vi "Run Bitfile velocity.vi"() -> ()   [LabVIEW 2011]
uses:
  <vilib>/Platform/TimedLoop/XDataNode/timing_clust.ctl
  <vilib>/Platform/TimedLoop/XDataNode/nitl_modes.ctl
  <vilib>/Platform/TimedLoop/XDataNode/wakeup.ctl
  <vilib>/FPGAPlugInAG/sbRIO-9606/niLvFpga_Open_sbRIO-9606.vi
  <vilib>/rvi/interface/common/dynamic/niFpgaDynamicAddResources.vi
  <vilib>/Utility/error.llb/Error Cluster From Error Code.vi
  <vilib>/rvi/errors/niLvFpgaAdjustHostInterfaceError.vi
  <vilib>/FPGAPlugInAG/Dynamic/niLvFpga_Close_Dynamic.vi
  <vilib>/Platform/TimedLoop/XDataNode/XDataNode.xnode
  <vilib>/rvi/interface/nirviOpenFPGA/nirviOpenFPGA.xnode
  labview/FPGA Bitfiles/natcar_FPGATarget_Top-Level_610FB000.lvbitx
  <vilib>/rvi/interface/nirviReadWriteControl/nirviReadWriteControl.xnode
  <vilib>/rvi/interface/nirviCloseFPGA/nirviCloseFPGA.xnode
  <vilib>/Platform/TimedLoop/XDataNode/XDNodeRunTimeDep.lvlib
  NiFpgaLv.dll
  <vilib>/rvi/interface/Simulation/niFpgaSimulationCallBeginRW.vi
panel:
  out "Speed Error":dbl(graph)
  in  "Offset":dbl=22.0 min=0.0 max=30.0 step=0.1
  out "Velocity counts":u32
  out "V [m/s]":dbl
  in  "RUN!":bool
  in  "Stop":bool
  in  "Kff":dbl=6.0 min=0.0 max=10.0 step=0.1
  in  "uBlaze Reset":bool
  in  "Steering ON 1e-7s":u32=15000 min=10240 max=19650 step=100
  in  "Steering":bool
  in  "Throttle":bool
  in  "GO frequency (Hz)":u16=1000 min=10 max=10000 step=10
  in  "GO duty (100*%)":u16 max=100 step=1
  in  "V desired [m/s]":dbl min=0.0 max=5.0 step=0.1
  in  "Speed Ki":dbl=0.1 min=0.0 max=2.0 step=0.01
  in  "Throttle ON":bool
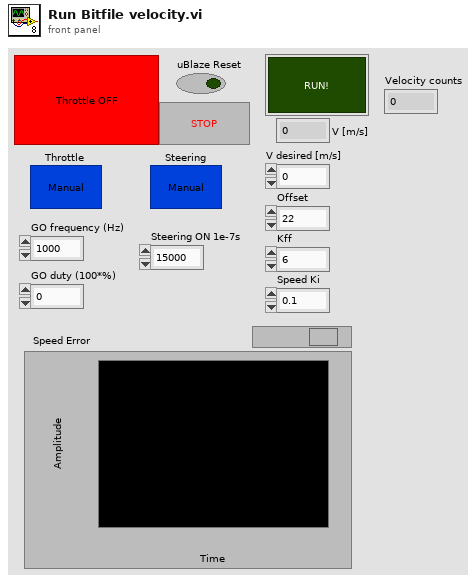
[diagram p1: front panel]
types:
  T1 = typedef "XDNodeRunTimeDep.lvlib/timing_clust.ctl" = cluster{"Expected End [f-1]":u64, "Actual End [f-1]":u64, "Finished Late? [f-1]":bool, "Expected End [i-1]":u64, "Actual End [i-1]":u64, "Finished Late? [i-1]":bool, "Expected Start [i]":u64, "Actual Start [i]":u64, "Expected Start [f]":u64, "Actual Start [f]":u64, "Source Name":string, "Structure Name":string, "Period":i64, "Deadline":i64, "Offset":i64, "Start":i64, "Priority":i32, "Timeout":i32, "Mode":T2, "Wakeup Reason":T3, "Error":errorcluster, "Source Type":string, "Secondary Source Type":string, "Global End Time":u64, "Global Start Time":u64, "Frame Duration":u64, "Iteration Duration":u64, "Assigned CPU":i32, "I/O Scan Engine Mode":u32}
  T2 = typedef "XDNodeRunTimeDep.lvlib/nitl_modes.ctl" = enum32{"No Change", "Process missed periods, maintain original phase", "Discard missed periods, maintain original phase", "Process missed periods, ignore original phase", "Discard missed periods, ignore original phase"}
  T3 = typedef "XDNodeRunTimeDep.lvlib/wakeup.ctl" = enum32{"Normal", "Aborted", "Asynchronous wakeup", "Timing source error", "Timed loop error", "Timeout"}
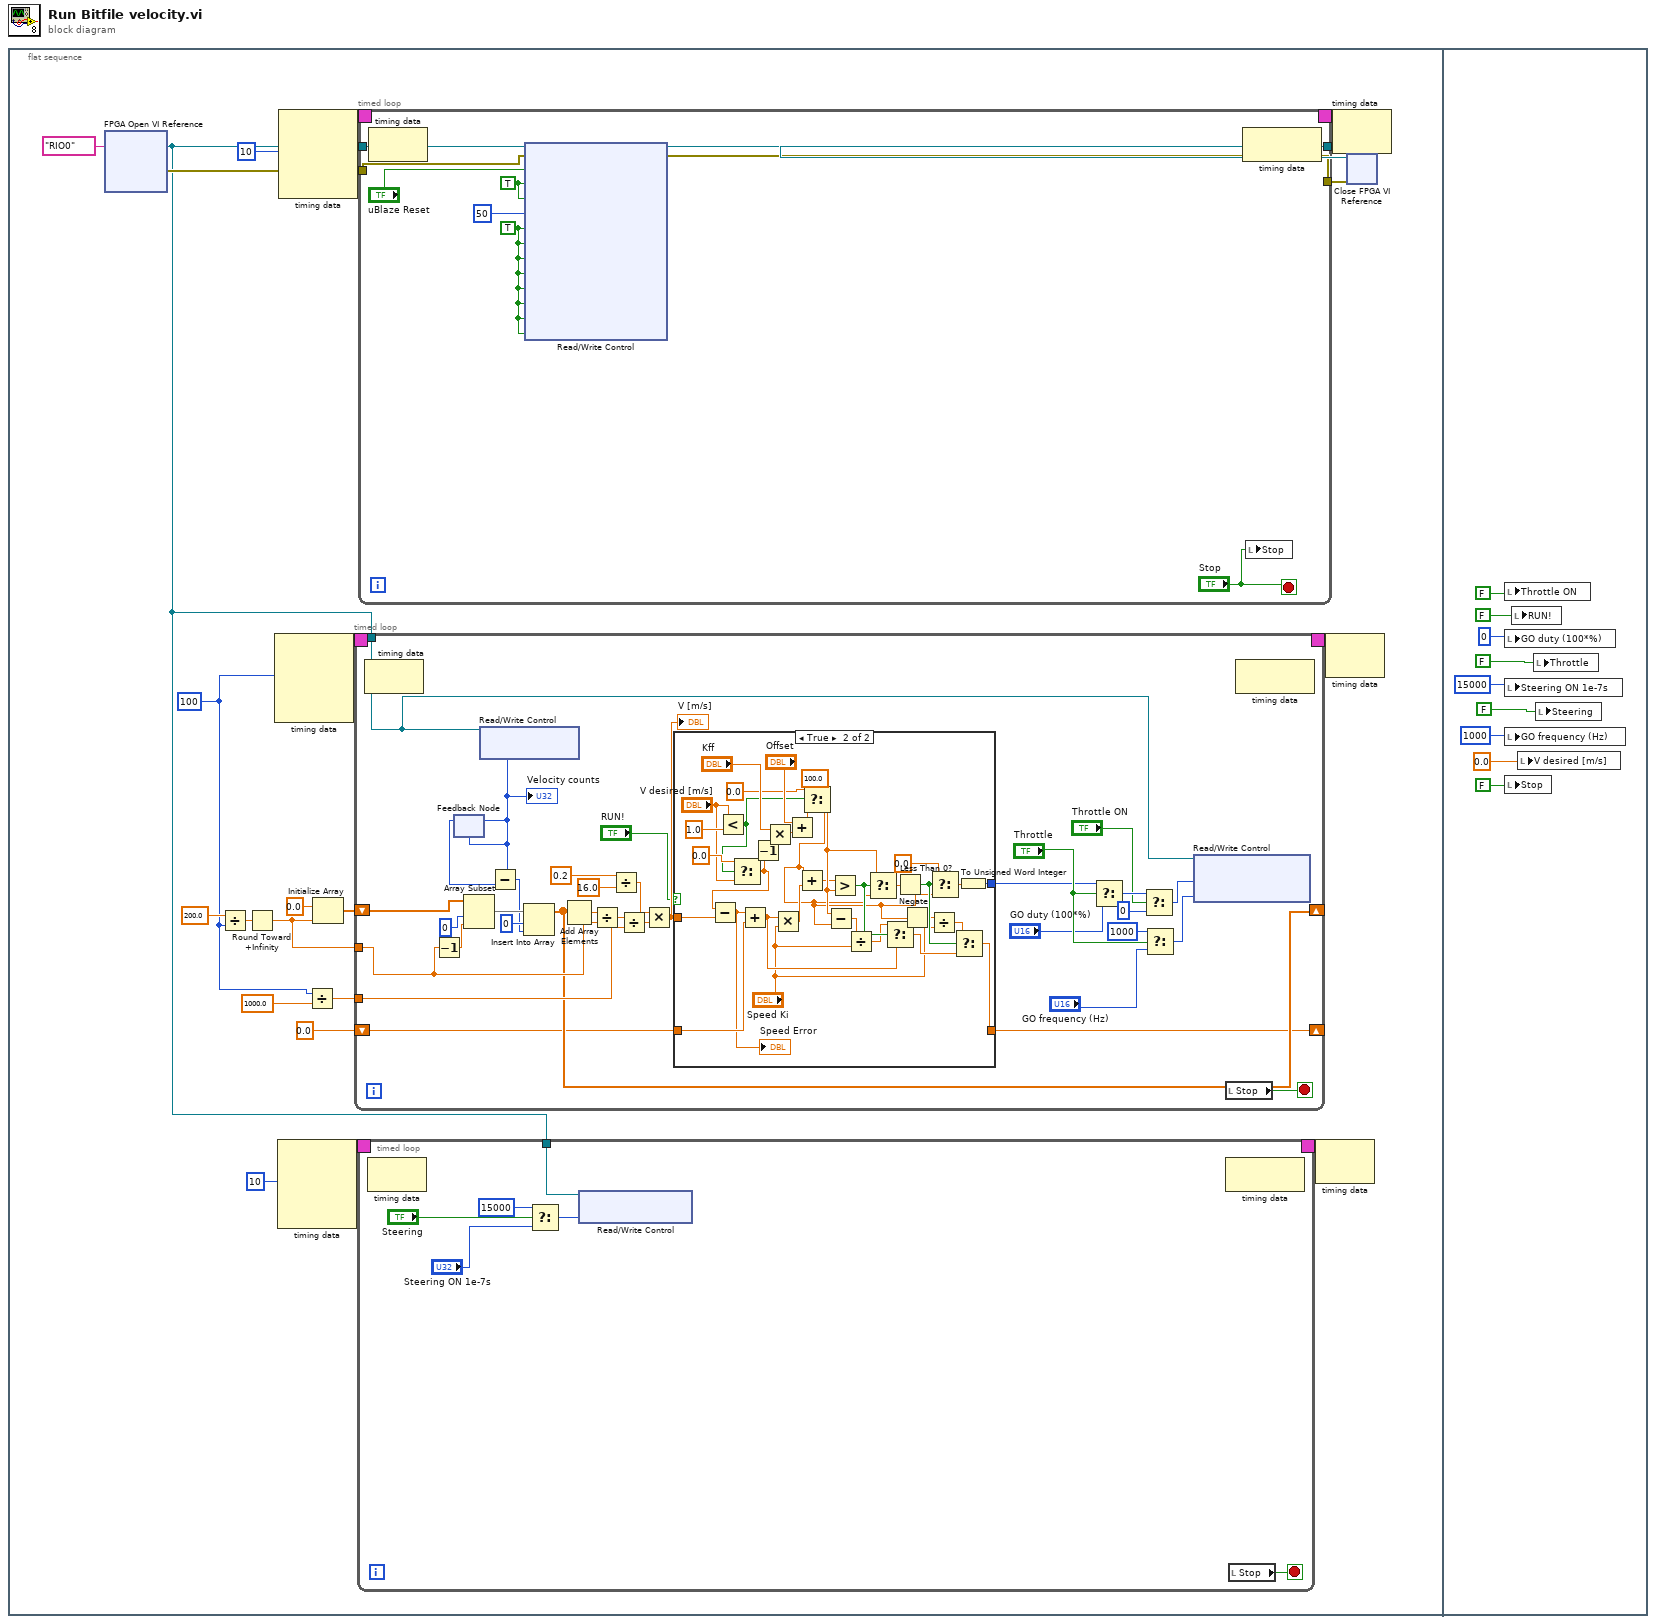
[diagram p0: block diagram]
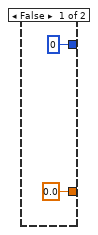
[diagram p2: hidden frame]
diagram:
  n1 = flat-sequence {
    frame #0 {
      w1 = i64 100 ("Period")
      n2 = xnode "FPGA Open VI Reference"("resource name"=tag "RIO0") -> ("FPGA VI Reference Out"=w4:refnum<k20>, "error out"=w15:errorcluster)  [unwired: 1 in]
      n3 = Divide(x=200.0, y=w1) -> (x/y=w9:dbl)
      n4 = Round Toward +Infinity(x=w9) -> (ceil(x): smallest int >= x=w8:dbl)
      n5 = node-c288(w1) -> (w22:T1)  [unwired: 3 in]
      n6 = node-c288(i64 10 ("Period")) -> (w20:T1)  [unwired: 3 in]
      n7 = node-c288(i64 10 ("Period")) -> (w18:T1)  [unwired: 3 in]
      n8 = Divide(x=w1, y=1000.0) -> (x/y=w3:dbl)
      n9 = Initialize Array(0.0 ("element"), w8) -> (w12:dbl[])
      n10 = timed-loop {
        timing: w22 -> [_]
        timing-out: [_] -> w21
        shift-right: [w80] -> _
        shift-left: w12 -> [w79]
        tunnel: w8 -> [w82]
        tunnel: w3 -> [w81]
        shift-right: [w77] -> _
        shift-left: 0.0 -> [w78]
        tunnel: w4 -> [w76]
        stop <- w75 stop-if-true
        n11 = node-c288() -> ()  [unwired: 1 in, 1 out]
        n12 = Decrement(x=w82) -> (x-1=w63:dbl)
        n13 = Array Subset(array=w79, index=0, length=w63) -> (w55:dbl[])
        n14 = xnode "Read/Write Control"("FPGA VI Reference In"=w76) -> ("Velocity counts"=w51:u32)  [unwired: 1 in, 2 out]
        "Velocity counts" <- w51
        n15 = feedback #1(w51) -> (w52:u32)
        n16 = feedback-in #1(w51) -> ()
        n17 = Subtract(x=w51, y=w52) -> (x-y=w54:u32)
        n18 = Insert Into Array(array=w55, index=0, new element=w54) -> (w80:dbl[])
        n19 = Add Array Elements(numeric array=w80) -> (sum=w53:dbl)
        n20 = Divide(x=w53, y=w82) -> (x/y=w61:dbl)
        n21 = Divide(x=0.2, y=16.0) -> (x/y=w57:dbl)
        n22 = Divide(x=w61, y=w81) -> (x/y=w58:dbl)
        n23 = Multiply(x=w57, y=w58) -> (x*y=w56:dbl)
        "V [m/s]" <- w56
        n24 = case shown="True" "RUN!" {
          tunnel: w78 -> [_ w116]
          tunnel: [0.0 w115] -> w77
          tunnel: [u16 0 w114] -> w70
          tunnel: w56 -> [_ w113]
          frame False {
          }
          frame True {
            w107 = 100.0 ("y")
            n25 = Less?(x="V desired [m/s]", y=1.0) -> (x < y?=w89:bool)
            n26 = Select(t=0.0, s=w89, f="V desired [m/s]") -> (s? t:f=w90:dbl)
            n27 = Subtract(x=w90, y=w113) -> (x-y=w85:dbl)
            "Speed Error" <- w85
            n28 = Add(x=w85, y=w116) -> (x+y=w100:dbl)
            n29 = Decrement(x=w90) -> (x-1=w91:dbl)
            n30 = Multiply(x="Kff", y=w91) -> (x*y=w94:dbl)
            n31 = Multiply(x=w100, y="Speed Ki") -> (x*y=w112:dbl)
            n32 = Add(x="Offset", y=w94) -> (x+y=w87:dbl)
            n33 = Select(t=0.0, s=w89, f=w87) -> (s? t:f=w86:dbl)
            n34 = Add(x=w86, y=w112) -> (x+y=w103:dbl)
            n35 = Subtract(x=w107, y=w86) -> (x-y=w106:dbl)
            n36 = Greater?(x=w103, y=w107) -> (0:w108:bool)
            n37 = Divide(x=w106, y="Speed Ki") -> (x/y=w105:dbl)
            n38 = Select(t=w107, s=w108, f=w86) -> (s? t:f=w109:dbl)
            n39 = Select(t=w105, s=w108, f=w100) -> (s? t:f=w98:dbl)
            n40 = Less Than 0?(x=w109) -> (x < 0?=w104:bool)
            n41 = Negate(x=w86) -> (-x=w102:dbl)
            n42 = Divide(x=w102, y="Speed Ki") -> (x/y=w101:dbl)
            n43 = Select(t=0.0, s=w104, f=w86) -> (s? t:f=w99:dbl)
            n44 = Select(t=w101, s=w104, f=w98) -> (s? t:f=w115:dbl)
            n45 = To Unsigned Word Integer(number=w99) -> (unsigned 16bit integer=w114:u16)
          }
        }
        n46 = Select(t=w70, s="Throttle", f="GO duty (100*%)") -> (s? t:f=w67:u16)
        n47 = Select(t=w67, s="Throttle ON", f=u16 0 ("t")) -> (s? t:f=w66:u16)
        n48 = Select(t=u16 1000, s="Throttle", f="GO frequency (Hz)") -> (s? t:f=w69:u16)
        n49 = xnode "Read/Write Control"("FPGA VI Reference In"=w76, "GO duty (100*%)"=w66, "GO frequency (Hz)"=w69) -> ()  [unwired: 1 in, 2 out]
        n50 = local read "Stop"() -> (w75:bool)
        n51 = node-c288() -> ()  [unwired: 1 in, 1 out]
      }
      n52 = timed-loop {
        timing: w20 -> [_]
        timing-out: [_] -> w19
        tunnel: w4 -> [w39]
        stop <- w38 stop-if-true
        n53 = node-c288() -> ()  [unwired: 1 in, 1 out]
        n54 = Select(t=u32 15000, s="Steering", f="Steering ON 1e-7s") -> (s? t:f=w43:u32)
        n55 = xnode "Read/Write Control"("FPGA VI Reference In"=w39, "Steering ON 1e-7s"=w43) -> ()  [unwired: 1 in, 2 out]
        n56 = node-c288() -> ()  [unwired: 1 in, 1 out]
        n57 = local read "Stop"() -> (w38:bool)
      }
      n58 = timed-loop {
        tunnel: w4 -> [w31]
        tunnel: [w30] -> w16
        tunnel: w15 -> [w28]
        tunnel: [w27] -> w14
        timing: w18 -> [_]
        timing-out: [_] -> w17
        stop <- "Stop" stop-if-true
        w23 = TRUE ("Enable AI0")
        w26 = TRUE ("manual steering")
        n59 = node-c288() -> ()  [unwired: 1 in, 1 out]
        n60 = xnode "Read/Write Control"("FPGA VI Reference In"=w31, "error in"=w28, "uBlaze Reset"="uBlaze Reset", "manual steering"=w26, "manual throttle"=w26, "Steering frequency (Hz)"=u16 50, "Enable AI0"=w23, "Enable AI1"=w23, "Enable AI2"=w23, "Enable AI3"=w23, "Enable AI4"=w23, "Enable AI5"=w23, "Enable AI6"=w23, "Enable AI7"=w23) -> ("FPGA VI Reference Out"=w30:refnum<k20>, "error out"=w27:errorcluster)
        n61 = node-c288() -> ()  [unwired: 1 in, 1 out]
        n62 = local write "Stop"("Stop") -> ()
      }
      n63 = node-c288(w19) -> ()  [unwired: 1 out]
      n64 = node-c288(w21) -> ()  [unwired: 1 out]
      n65 = node-c288(w17) -> ()  [unwired: 1 out]
      n66 = xnode "Close FPGA VI Reference"("FPGA VI Reference In"=w16, "error in"=w14) -> ()  [unwired: 1 out]
    }
    frame #1 {
      n67 = local write "Throttle ON"(FALSE ("Throttle ON")) -> ()
      n68 = local write "GO duty (100*%)"(u16 0 ("GO duty (100*%)")) -> ()
      n69 = local write "Steering ON 1e-7s"(u32 15000 ("Steering ON 1e-7s")) -> ()
      n70 = local write "GO frequency (Hz)"(u16 1000 ("GO frequency (Hz)")) -> ()
      n71 = local write "Stop"(FALSE ("Stop")) -> ()
      n72 = local write "RUN!"(FALSE ("START!")) -> ()
      n73 = local write "V desired [m/s]"(0.0 ("Desired Speed [m/s]")) -> ()
      n74 = local write "Throttle"(FALSE ("Automatic Throttle")) -> ()
      n75 = local write "Steering"(FALSE ("Automatic Steering")) -> ()
    }
  }
